vi "Configure Timing.vi"(8 "error in":errorcluster, 11 "DAQmx Base CFG in":refnum<class "DAQmx Base CFG.lvclass">) -> (0 "error out":errorcluster, 3 "DAQmx Base CFG out":refnum<class "DAQmx Base CFG.lvclass">)   [LabVIEW 2023, in "DAQmx Base CFG.lvclass"]
uses:
  DAQmx Base CFG.lvclass
  Configurations/CFG Base/CFG Base.lvclass/CFG Base.ctl
  DAQmx Base CFG.lvclass/DAQmx Base CFG.ctl
  3a10eacc-4dca-40d5-9fc9-a43ea3856a05.vi
  <vilib>/JDP Science/JSONtext/Find Item.vi
  <vilib>/JDP Science/JSONtext/Next JSON Value.vi
  <vilib>/JDP Science/JSONtext/String Subset.vi
  <vilib>/JDP Science/JSONtext/Parsing/Advance past next JSON Value (inlined COPY).vi
  <vilib>/JDP Science/JSONtext/Parsing/Advance past whitespace.vi
  <vilib>/JDP Science/JSONtext/Parsing/Advance past String.vi
  <vilib>/JDP Science/JSONtext/Parsing/Advance past Number.vi
  <vilib>/JDP Science/JSONtext/Parsing/Advance past Line Ending.vi
  <vilib>/JDP Science/JSONtext/Parsing/Parse Full Path or Item Name.vi
  <vilib>/JDP Science/JSONtext/Parsing/Advance past Array.vi
  <vilib>/JDP Science/JSONtext/Parsing/Advance past Object.vi
  <vilib>/JDP Science/JSONtext/support/Error Cluster From Code.vi
  <vilib>/JDP Science/JSONtext/Offset/Find Item Locations by Path.vi
  <vilib>/JDP Science/JSONtext/JSON text to Variant.vi
  <vilib>/Utility/error.llb/Error Cluster From Error Code.vi
  <vilib>/DAQmx/configure/timing.llb/DAQmx Timing (Sample Clock).vi
  <vilib>/DAQmx/configure/timing.llb/DAQmx Timing (Implicit).vi
  <vilib>/JDP Science/JSONtext/LVClass Serializer/JSONtext LVClass Serializer.lvclass
  <vilib>/ErrorRing/Error Ring.xnode
  Configurations/CFG JSON/CFG JSON.lvclass
  Configurations/CFG Base/CFG Base.lvclass
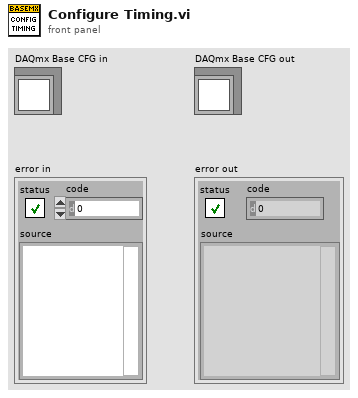
[diagram p1: front panel]
types:
  T1 = cluster{"Type":string, "Samples per Channel":i32, "Sample Mode":string, "Sample Rate":dbl, "Sample Clock Source":string, "Active Edge":string}
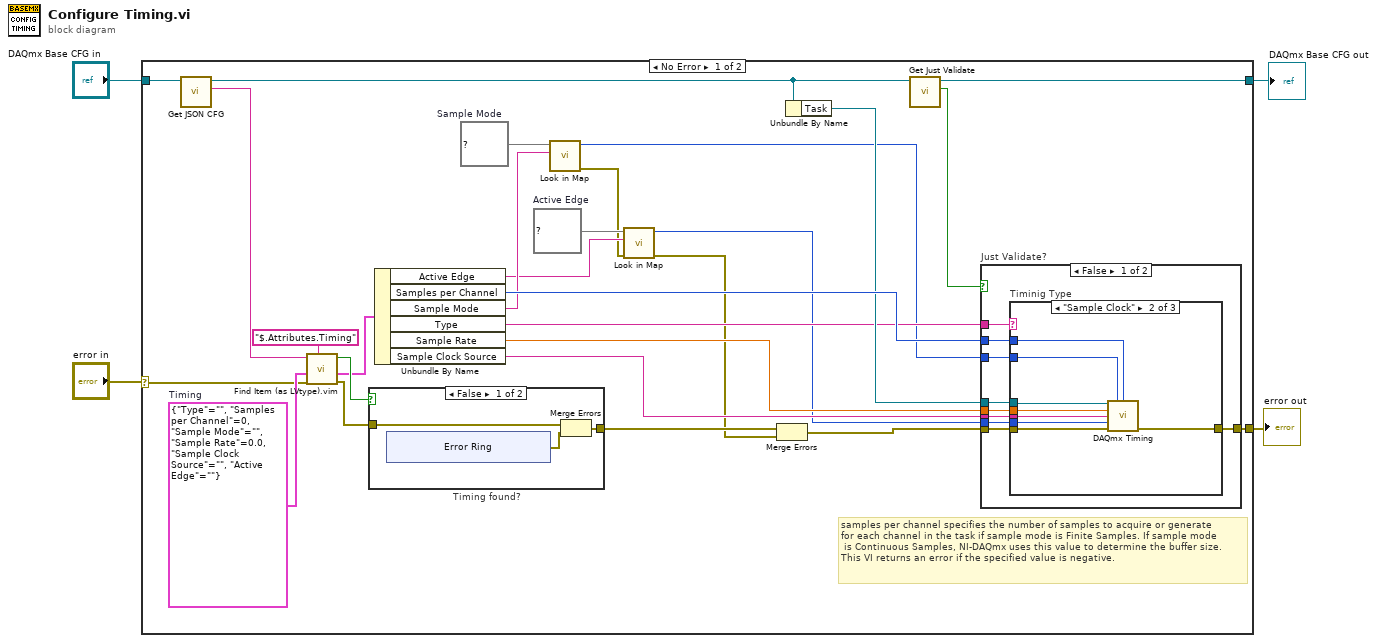
[diagram p0: block diagram]
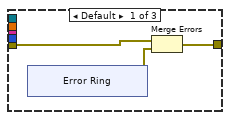
[diagram p2: hidden frame]
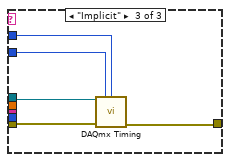
[diagram p3: hidden frame]
diagram:
  n1 = case shown="No Error" "error in" {
    selector: "error in" -> [w14 w73]
    tunnel: [w20 w73] -> w4
    tunnel: "DAQmx Base CFG in" -> [w19 w72]
    tunnel: [w18 w72] -> w2
    frame No Error {
      w9 = map{string, i32} {"Falling"=10171, "Rising"=10280}  # Active Edge
      w12 = map{string, i32} {"Continuous Samples"=10123, "Finite Samples"=10178, "Hardware Timed Single Point"=12522}  # Sample Mode
      w29 = T1 {"Type"="", "Samples per Channel"=0, "Sample Mode"="", "Sample Rate"=0.0, "Sample Clock Source"="", "Active Edge"=""}  # Timing
      # "samples per channel specifies the number of samples to acquire or generate\nfor each channel in the task if sample mode is Finite Samples. If sample mode\n is Continuous Samples, NI-DAQmx uses this value to determine the buffer size.\nThis VI returns an error if the specified value is negative."
      n2 = call "Get JSON CFG.vi"("CFG JSON in"=w19) -> ("<JSON> CFG"=w31:string, "CFG JSON out"=w13:refnum<class "DAQmx Base CFG.lvclass">)  [unwired: 9 in]
      n3 = call "Find Item (as LVtype).vim"("$Path or Item Name"="$.Attributes.Timing", "error in (no error)"=w14, "Data Type and Default Value"=w29, "JSON"=w31) -> ("error out"=w27:errorcluster, "Data"=w26:T1, "Found"=w28:bool)  [unwired: 4 in, 1 out]
      n4 = case "Timing found?" shown="False" w28 {
        tunnel: w27 -> [w64 w71]
        tunnel: [w63 w71] -> w25
        frame False {
          n5 = xnode "Error Ring"() -> ("error out"=w65:errorcluster)
          n6 = Merge Errors(w64, w65) -> (w63:errorcluster)
        }
        frame True {
        }
      }
      n7 = Unbundle By Name(w26) -> ("Active Edge"=w8:string, "Samples per Channel"=w22:i32, "Sample Mode"=w11:string, "Type"=w16:string, "Sample Rate"=w23:dbl, "Sample Clock Source"=w24:string)
      n8 = call "Look in Map.vi"("Key"=w11, "Map"=w12) -> ("error out"=w7:errorcluster, "Value"=w10:i32)  [unwired: 8 in]
      n9 = call "Look in Map.vi"("error in"=w7, "Key"=w8, "Map"=w9) -> ("error out"=w6:errorcluster, "Value"=w5:i32)  [unwired: 7 in]
      n10 = Merge Errors(w25, w6) -> (w15:errorcluster)
      n11 = Unbundle By Name(w13) -> ("Task"=w21:refnum<k21>)
      n12 = call "Get Just Validate.vi"("CFG Base in"=w13) -> ("Just Validate"=w17:bool, "CFG Base out"=w18:refnum<class "DAQmx Base CFG.lvclass">)  [unwired: 9 in]
      n13 = case "Just Validate?" shown="False" w17 {
        tunnel: w15 -> [w40 w62]
        tunnel: w24 -> [w39 _]
        tunnel: w23 -> [w38 _]
        tunnel: w10 -> [w37 _]
        tunnel: w22 -> [w36 _]
        tunnel: w21 -> [w35 _]
        tunnel: w5 -> [w34 _]
        tunnel: [w33 w62] -> w20
        tunnel: w16 -> [w32 _]
        frame False {
          n14 = case "Timinig Type" shown="\"Sample Clock\"" w32 {
            tunnel: w40 -> [w42 w56 w59]
            tunnel: w39 -> [_ w55 _]
            tunnel: w38 -> [_ w54 _]
            tunnel: w37 -> [_ w53 w58]
            tunnel: w36 -> [_ w52 w57]
            tunnel: w35 -> [_ w51 w60]
            tunnel: [w43 w50 w61] -> w33
            tunnel: w34 -> [_ w49 _]
            frame Default {
              n15 = xnode "Error Ring"() -> ("error out"=w41:errorcluster)
              n16 = Merge Errors(w42, w41) -> (w43:errorcluster)
            }
            frame "Sample Clock" {
              n17 = call-poly <vilib>:"DAQmx Timing.vi"("task/channels in"=w51, "sample mode"=w53, "samples per channel"=w52, "rate"=w54, "source"=w55, "active edge"=w49, "error in"=w56) -> ("error out"=w50:errorcluster)  [unwired: 7 in, 1 out]
            }
            frame "Implicit" {
              n18 = call-poly <vilib>:"DAQmx Timing.vi"("task/channels in"=w60, "sample mode"=w58, "samples per channel"=w57, "error in"=w59) -> ("error out"=w61:errorcluster)  [unwired: 10 in, 1 out]
            }
          }
        }
        frame True {
        }
      }
    }
    frame Error {
    }
  }
  "error out" <- w4
  "DAQmx Base CFG out" <- w2
